vi "Date and Time.vi"() -> (3 "Current Time":string)   [LabVIEW 2021, in "User Interface.lvlib"]
uses:
  User Interface.lvlib
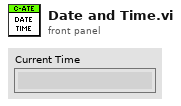
[diagram p1: front panel]
types:
  T1 = typedef "LVDateTimeRec.ctl" = cluster{"fractional second":dbl, "second":i32, "minute":i32, "hour":i32, "day of month":i32, "month":i32, "year":i32, "day of week":i32, "day of year":i32, "DST":i32}
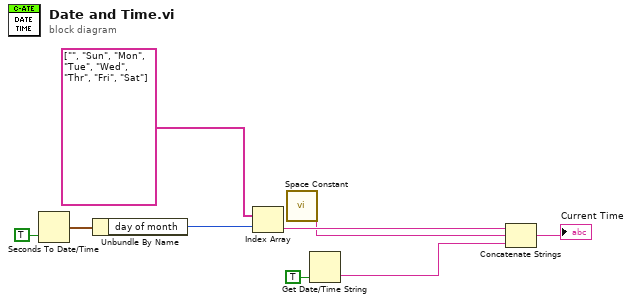
[diagram p0: block diagram]
diagram:
  n1 = Seconds To Date/Time(to UTC (F)=TRUE) -> (date time rec=w8:T1)  [unwired: 1 in]
  n2 = Unbundle By Name(w8) -> ("day of month"=w6:i32)
  n3 = Index Array(array=string[] ["", "Sun", "Mon", "Tue", "Wed", "Thr", "Fri", "Sat"], index=w6) -> (element=w5:string)
  n4 = call <vilib>:"Space Constant.vi"() -> ("String"=w4:string)
  n5 = Get Date/Time String(want seconds? (F)=TRUE) -> (time string=w1:string)  [unwired: 2 in, 1 out]
  n6 = Concatenate Strings(w5, w4, w1) -> (→"Current Time":string)
